vi "Create Sysdef Tree Labels.vi"(6 "first call":bool, 8 "error in":errorcluster, 9 "Labels":T2[](array[typedef]), 10 "Section Ptr":T1 format="%.0x", 11 "direction":T6(ring)) -> (0 "error out":errorcluster)   [LabVIEW 2011, in "AIT 429 Custom Device.lvlib"]
uses:
  AIT 429 Custom Device.lvlib
  Controls/AIT_Label.ctl
  Controls/AIT_Word.ctl
  Controls/ARINCParam.ctl
  Controls and Global/TransferType.ctl
  <vilib>/NI Veristand/Custom Device API/Custom Device Item Ref.ctl
  <vilib>/NI Veristand/Custom Device API/Custom Device Channel.ctl
  <vilib>/NI Veristand/Custom Device API/Custom Device Channel Type.ctl
  Controls and Global/Global.vi
  <vilib>/NI Veristand/Custom Device API/Custom Device API.lvlib
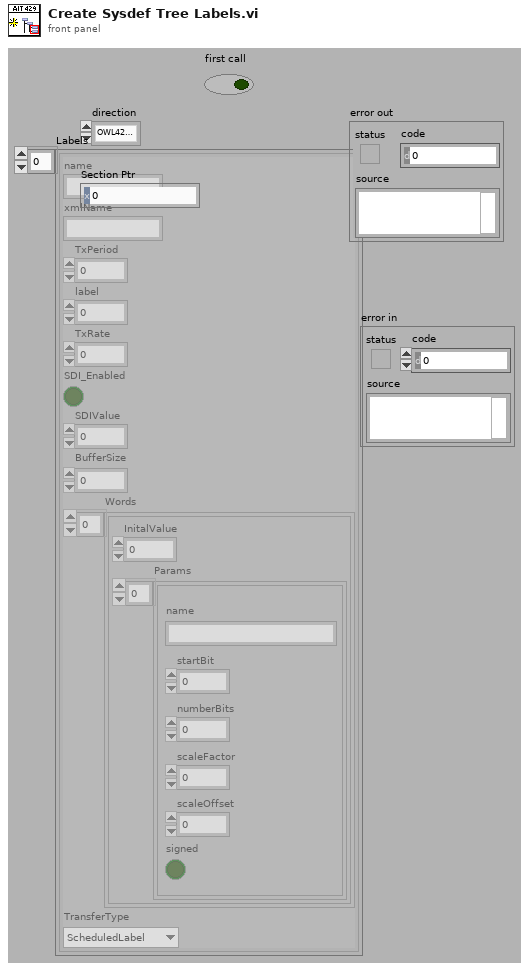
[diagram p1: front panel]
types:
  T1 = typedef "Custom Device API.lvlib/Custom Device Item Ref.ctl" = u64
  T2 = typedef "AIT 429 Custom Device.lvlib/AIT_Label.ctl" = cluster{"name":string, "xmlName":string, "TxPeriod":u32, "label":u32, "TxRate":dbl, "SDI_Enabled":bool, "SDIValue":u8, "BufferSize":u32, "Words":T3[], "TransferType":T5}
  T3 = typedef "AIT 429 Custom Device.lvlib/AIT_Word.ctl" = cluster{"InitalValue":u32, "Params":T4[]}
  T4 = typedef "AIT 429 Custom Device.lvlib/ARINCParam.ctl" = cluster{"name":string, "startBit":i32, "numberBits":i32, "scaleFactor":dbl, "scaleOffset":dbl, "signed":bool}
  T5 = typedef "AIT 429 Custom Device.lvlib/TransferType.ctl" = enum16{"ScheduledLabel", "Acyclic", "Block", "Strobe"}
  T6 = enum16{"OWL429_DIRECTION_RX", "OWL429_DIRECTION_TX"}
  T7 = typedef "Custom Device API.lvlib/Custom Device Channel.ctl" = cluster{"Type":T8, "Units":string, "Default Value":dbl, "Faultable":bool, "Scalable":bool}
  T8 = typedef "Custom Device API.lvlib/Custom Device Channel Type.ctl" = enum16{"Input", "Output"}
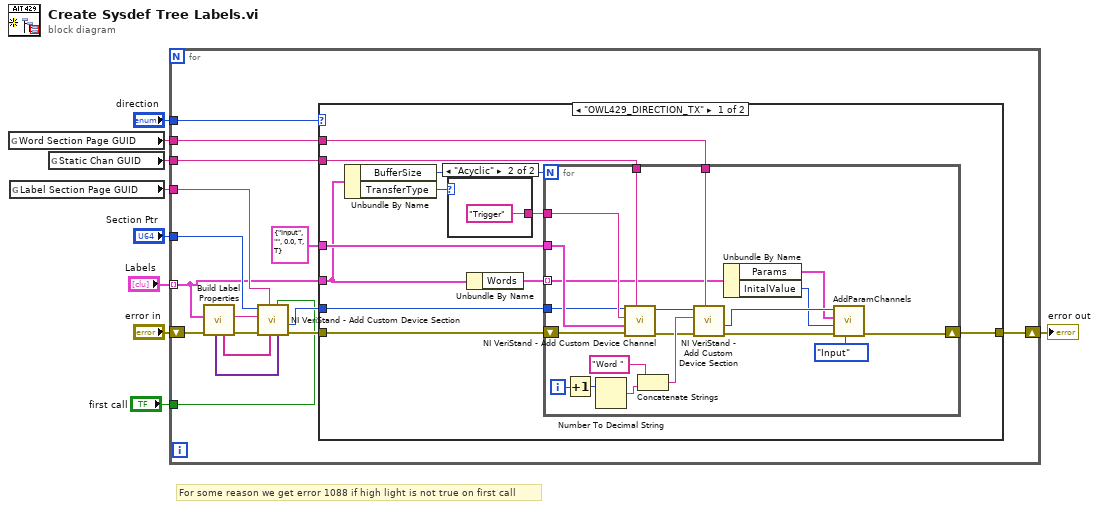
[diagram p0: block diagram]
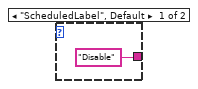
[diagram p2: hidden frame]
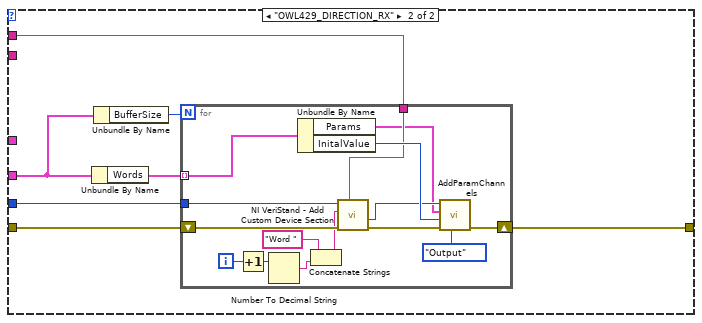
[diagram p3: hidden frame]
diagram:
  # "For some reason we get error 1088 if high light is not true on first call"
  n1 = global read "Global.vi" "Word Section Page GUID"() -> (w4:string)
  n2 = global read "Global.vi" "Label Section Page GUID"() -> (w6:string)
  n3 = global read "Global.vi" "Static Chan GUID"() -> (w5:string)
  n4 = for {
    shift-right: [w22] -> w3
    shift-left: "error in" -> [w14]
    tunnel: "Section Ptr" -> [w24]
    tunnel: "Labels" -> [w16] mode=indexing
    tunnel: "direction" -> [w21]
    tunnel: w6 -> [w19]
    tunnel: w5 -> [w18]
    tunnel: w4 -> [w15]
    tunnel: "first call" -> [w10]
    n5 = call "Build Label Properties.vi"("error in (no error)"=w14, "Labels"=w16) -> ("error out"=w13:errorcluster, "name"=w11:string, "Prop Names"=w23:string[], "Prop Values"=w25:variant[])  [unwired: 6 in]
    n6 = call <vilib>:"NI VeriStand - Add Custom Device Section.vi"("Property Values"=w25, "Highlight? (F)"=w10, "Property names"=w23, "GUID (Default Section)"=w19, "error in (no error)"=w13, "Section Name"=w11, "Parent Ref in"=w24) -> ("error out"=w12:errorcluster, "Section Ptr"=w17:T1)  [unwired: 1 in, 2 out]
    n7 = case shown="\"OWL429_DIRECTION_TX\"" w21 {
      tunnel: w12 -> [w33 w65]
      tunnel: w17 -> [w32 w62]
      tunnel: [w36 w64] -> w22
      tunnel: T7 {"Type"=enum."Input", "Units"="", "Default Value"=0.0, "Faultable"=TRUE, "Scalable"=TRUE} ("Channel") -> [w35 _]
      tunnel: w18 -> [w34 _]
      tunnel: w16 -> [w29 w63]
      tunnel: w15 -> [w31 w61]
      frame "OWL429_DIRECTION_TX" {
        n8 = Unbundle By Name(w29) -> ("BufferSize"=w28:u32, "TransferType"=w27:T5)
        n9 = case shown="\"Acyclic\"" w27 {
          tunnel: ["Disable" ("Channel Name") "Trigger" ("Static Chan GUID")] -> w26
          frame "ScheduledLabel", Default {
          }
          frame "Acyclic" {
          }
        }
        n10 = Unbundle By Name(w29) -> ("Words"=w30:T3[])
        n11 = for {
          N: w28 -> [_]
          tunnel: w35 -> [w58]
          tunnel: w26 -> [w57]
          tunnel: w34 -> [w56]
          tunnel: w32 -> [w49]
          tunnel: w30 -> [w46] mode=indexing
          shift-right: [w42] -> w36
          shift-left: w33 -> [w48]
          tunnel: w31 -> [w51]
          i -> [w53]
          n12 = Increment(x=w53) -> (x+1=w54:i32)
          n13 = Number To Decimal String(number=w54) -> (decimal integer string=w55:string)  [unwired: 1 in]
          n14 = call <vilib>:"NI VeriStand - Add Custom Device Channel.vi"("GUID (Default Channel)"=w56, "error in (no error)"=w48, "Channel"=w58, "Channel Name"=w57, "Parent Ref in"=w49) -> ("error out"=w40:errorcluster, "Parent Ref out"=w47:T1)  [unwired: 3 in, 2 out]
          n15 = Concatenate Strings("Word " ("string"), w55) -> (w50:string)
          n16 = call <vilib>:"NI VeriStand - Add Custom Device Section.vi"("GUID (Default Section)"=w51, "error in (no error)"=w40, "Section Name"=w50, "Parent Ref in"=w47) -> ("error out"=w41:errorcluster, "Section Ptr"=w45:T1)  [unwired: 4 in, 2 out]
          n17 = Unbundle By Name(w46) -> ("Params"=w39:T4[], "InitalValue"=w44:u32)
          n18 = call "AddParamChannels.vi"("Type"=Custom_Device_Channel_Type."Input", "error in"=w41, "Initial Value"=w44, "Parameters to add"=w39, "Node Ref In"=w45) -> ("error out"=w42:errorcluster)  [unwired: 5 in, 1 out]
        }
      }
      frame "OWL429_DIRECTION_RX" {
        n19 = Unbundle By Name(w63) -> ("Words"=w60:T3[])
        n20 = Unbundle By Name(w63) -> ("BufferSize"=w59:u32)
        n21 = for {
          N: w59 -> [_]
          tunnel: w62 -> [w78]
          tunnel: w60 -> [w79] mode=indexing
          shift-right: [w66] -> w64
          shift-left: w65 -> [w77]
          tunnel: w61 -> [w75]
          i -> [w74]
          n22 = Increment(x=w74) -> (x+1=w72:i32)
          n23 = Number To Decimal String(number=w72) -> (decimal integer string=w71:string)  [unwired: 1 in]
          n24 = Unbundle By Name(w79) -> ("Params"=w67:T4[], "InitalValue"=w80:u32)
          n25 = Concatenate Strings("Word " ("string"), w71) -> (w73:string)
          n26 = call <vilib>:"NI VeriStand - Add Custom Device Section.vi"("GUID (Default Section)"=w75, "error in (no error)"=w77, "Section Name"=w73, "Parent Ref in"=w78) -> ("error out"=w76:errorcluster, "Section Ptr"=w68:T1)  [unwired: 4 in, 2 out]
          n27 = call "AddParamChannels.vi"("Type"=Custom_Device_Channel_Type."Output", "error in"=w76, "Initial Value"=w80, "Parameters to add"=w67, "Node Ref In"=w68) -> ("error out"=w66:errorcluster)  [unwired: 5 in, 1 out]
        }
      }
    }
  }
  "error out" <- w3
